vi "In Place Write 1D Array SGL.vi"(8 "error in (no error)":errorcluster, 9 "start index (0)":i64, 10 "values in":sgl[](array[numeric]), 11 "pointer in":u64) -> (0 "error out":errorcluster, 1 "start index out":i64, 2 "values out":sgl[](array[numeric]), 3 "pointer out":u64)   [LabVIEW 2013, in "Linux RT IPC.Shared Memory.lvlib"]
uses:
  Linux RT IPC.Shared Memory.lvlib
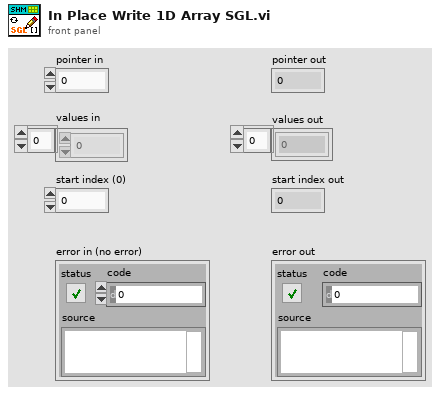
[diagram p1: front panel]
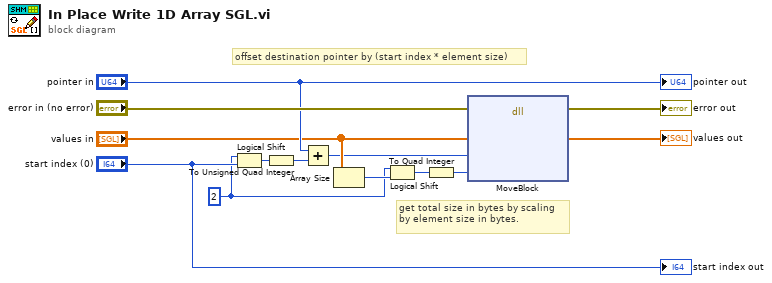
[diagram p0: block diagram]
diagram:
  w1 = i16 2 ("y")
  # "get total size in bytes by scaling by element size in bytes."
  # "offset destination pointer by (start index * element size)"
  n1 = Logical Shift(y=w1, x="start index (0)") -> (x << y=w6:i64)
  n2 = To Unsigned Quad Integer(1:w6) -> (0:w7:u64)
  n3 = Add(x="pointer in", y=w7) -> (x+y=w3:u64)
  n4 = Array Size(array="values in") -> (size(s)=w2:i32)
  n5 = Logical Shift(y=w1, x=w2) -> (x << y=w5:i32)
  n6 = To Quad Integer(1:w5) -> (0:w4:i64)
  n7 = dll-call lib="LabVIEW" fn="MoveBlock"(error in="error in (no error)", "data"="values in", "pointer"=w3, "size"=w4) -> (error out=→"error out":errorcluster, "data"=→"values out":sgl[])  [unwired: 5 in, 1 out]
  "pointer out" <- "pointer in"
  "start index out" <- "start index (0)"
